vi "T7MOD_Write_FLOAT32_Registers.vi"(7 "FLOAT32 to Write":sgl[](array[numeric]), 8 "error in":errorcluster, 9 "Starting FLOAT32 Register":i32=55124, 10 "Remote Port":u16=502, 11 "Remote IP Address":string="192.168.1.15") -> (0 "error out":errorcluster, 1 "Written At":timestamp)   [LabVIEW 2016]
uses:
  Serial Link Layer/NI_Modbus_Cleaned/NI Modbus121Clean.llb/MB Ethernet Master Query Write Multiple Registers (poly).vi
panel:
  # "Output"
  # "TCP Parameters"
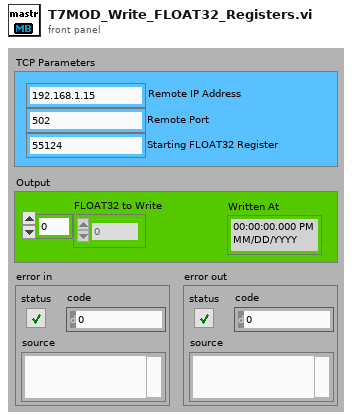
[diagram p1: front panel]
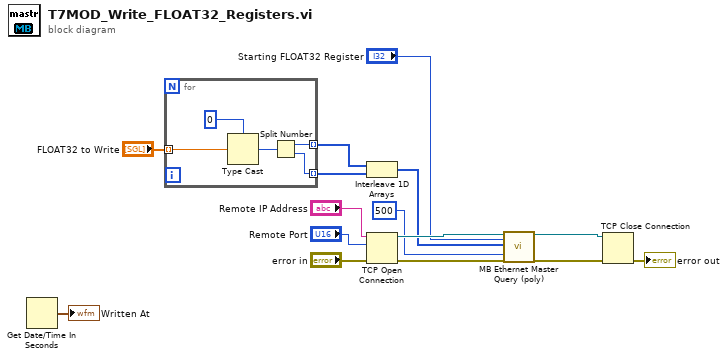
[diagram p0: block diagram]
diagram:
  n1 = Get Date/Time In Seconds() -> (seconds since 1Jan1904=→"Written At":timestamp)
  n2 = for {
    tunnel: [w20] -> w4 mode=indexing
    tunnel: [w19] -> w3 mode=indexing
    tunnel: "FLOAT32 to Write" -> [w17] mode=indexing
    n3 = Type Cast(type=u32 0, x=w17) -> (*(type *) &x=w16:u32)
    n4 = Split Number(x=w16) -> (hi(x)=w19:u16, lo(x)=w20:u16)
  }
  n5 = Interleave 1D Arrays(w3, w4) -> (w1:u16[])
  n6 = TCP Open Connection(address="Remote IP Address", remote port or service name="Remote Port", error in (no error)="error in") -> (connection ID=w13:refnum<k5>, error out=w12:errorcluster)  [unwired: 2 in]
  n7 = call-poly "MB Ethernet Master Query (poly).vi"("TCP Connection Refnum in"=w13, "Starting Address"="Starting FLOAT32 Register", "Registers"=w1, "Timeout"=500, "error in"=w12) -> ("TCP Connection Refnum (dup)"=w10:refnum<k5>, "error out"=w11:errorcluster)  [unwired: 12 in, 1 out]
  n8 = TCP Close Connection(connection ID=w10, error in (no error)=w11) -> (error out=→"error out":errorcluster)  [unwired: 2 out]
